vi "ATSh_Triggered.vi"(11 "Handle":u32) -> (0 "Return Code":u32, 2 "Triggered":bool, 3 "Handle_Out":u32)   [LabVIEW 2010]
doc: "_____AlazarTech, Scope_____\n\nQuery the devices's triggered status.\nHandle input."
uses:
  ATSApi.dll
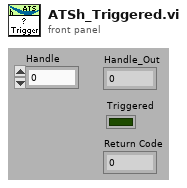
[diagram p1: front panel]
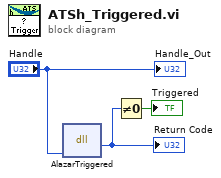
[diagram p0: block diagram]
diagram:
  n1 = dll-call lib="ATSApi.dll" fn="AlazarTriggered"("h"="Handle") -> (w2:u32)  [unwired: 4 in, 2 out]
  "Return Code" <- w2
  n2 = Not Equal To 0?(x=w2) -> (x != 0?=→"Triggered":bool)
  "Handle_Out" <- "Handle"
